vi "CODMn停止命令 (子VI).vi"   [LabVIEW 2016, in "斯坦道CODMn.lvlib"]
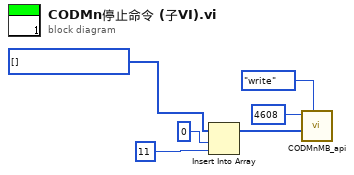
[diagram p0: block diagram]
diagram:
  n1 = Insert Into Array(array=u16[] [] ("values"), index=0 ("索引"), new element=u16 11 ("address")) -> (w2:u16[])
  n2 = call "CODMnMB_api.vi"("STEP"=enum16{"open", "read", "write", "close"}."write", "values"=w2, "starting address"=u16 4608 ("address")) -> ()  [unwired: 5 in, 4 out]
